vi "Vertical Profile.vi"(5 "Vert.Z-Locations":dbl[](array[numeric])=[12.7, 19.05, 25.4], 6 "Averaging time (min)":dbl, 7 "Starting Coords":T1={"X"=-100.0, "Y"=-150.0, "Z0"=45.0, "Name"="Anemo1"}, 10 "Tunnel Speed":dbl, 11 "Input Task Array":T4(array[cluster])) -> (3 "Output Task Array":T4(array[cluster]))   [LabVIEW 2015]
uses:
  Anemometry Sub Vis/Gen Trav/Spacing.ctl
  Anemometry Sub Vis/Controls/Multi_run_mode.ctl
  MRCMDFBGlobal.vi
  Set ADAM Ch.vi
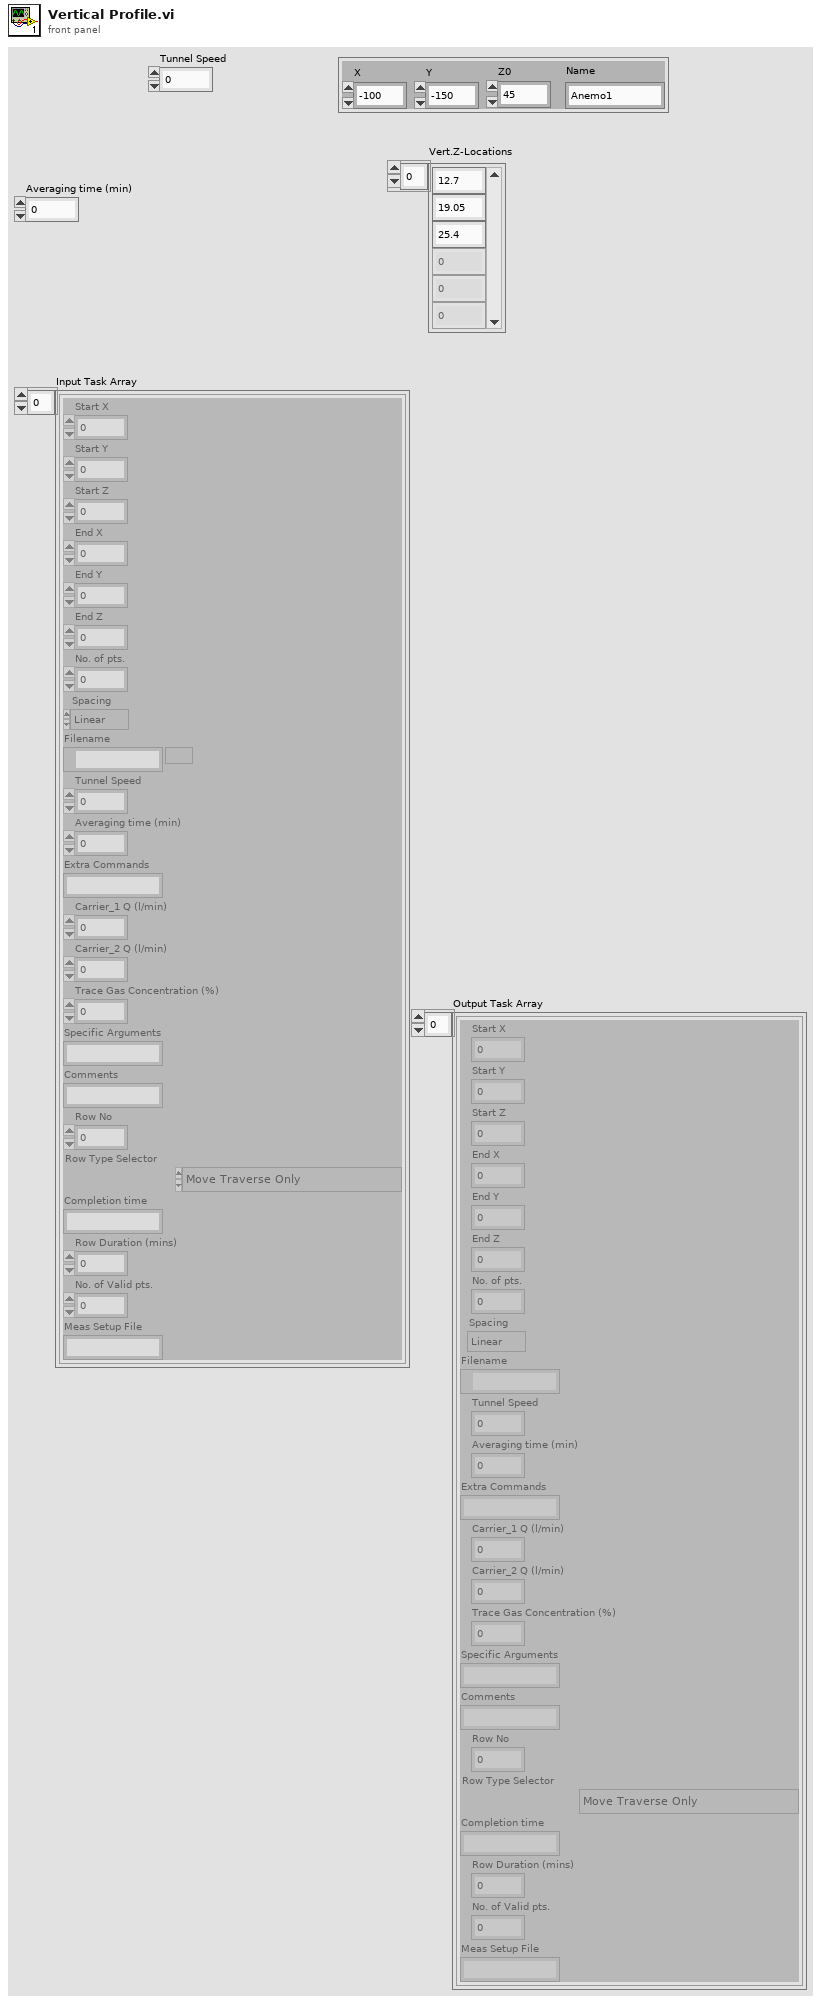
[diagram p1: front panel]
types:
  T1 = cluster{"X":dbl, "Y":dbl, "Z0":dbl, "Name":string}
  T2 = typedef "Spacing.ctl" = enum16{"Linear", "Log", "Gauss", "Specified", "N/A"}
  T3 = typedef "Multi_run_mode.ctl" = enum16{"Move Traverse Only", "Set Tunnel Speed Only", "Set Source Only", "Set Measurement Conditions", "Single Measurement", "Vertical Profile", "Lateral Profile", "Longitudinal Profile", "Explore Volume", "Multi-Axis Profile", "Auto Calibrate", "Meas Fast FID Bkgnd", "Check Beam Power", "Scanning Valve Measurement", "Run VI Named:", "Set ADAM Ch", "Wait (minutes)", "Send Message", "Synchronize With:", "Fall Back to this Row", "Turn Off Row Repeating", "Blank Row", "Traverse 3D Volume"}
  T4 = cluster{"Start X":sgl, "Start Y":sgl, "Start Z":sgl, "End X":sgl, "End Y":sgl, "End Z":sgl, "No. of pts.":i32, "Spacing":T2, "Filename":path, "Tunnel Speed":dbl, "Averaging time (min)":dbl, "Extra Commands":string, "Carrier_1 Q (l/min)":dbl, "Carrier_2 Q (l/min)":dbl, "Trace Gas Concentration (%)":dbl, "Specific Arguments":string, "Comments":string, "Row No":i32, "Row Type Selector":T3, "Completion time":string, "Row Duration (mins)":dbl, "No. of Valid pts.":i32, "Meas Setup File":string}[]
  T5 = cluster{"Start X":sgl, "Start Y":sgl, "Start Z":sgl, "End X":sgl, "End Y":sgl, "End Z":sgl, "No. of pts.":i32, "Spacing":T2, "Filename":path, "Tunnel Speed":dbl, "Averaging time (min)":dbl, "Extra Commands":string, "Carrier_1 Q (l/min)":dbl, "Carrier_2 Q (l/min)":dbl, "Trace Gas Concentration (%)":dbl, "Specific Arguments":string, "Comments":string, "Row No":i32, "Row Type Selector":T3, "Completion time":string, "Row Duration (mins)":dbl, "No. of Valid pts.":i32, "Meas Setup File":string}
  T6 = cluster{"Azimuth Array Index":u32, "Vert Prof Array Index":u32, "Lat Prof Array Index":u32, "Long Prof Array Index":u32}
  T7 = cluster{"TT.Azimuths":dbl[], "Z.HeightCorrs":dbl[][], "Use Height Corrections":bool, "Height Survey Filepaths":path[], "Corrections from File":bool}
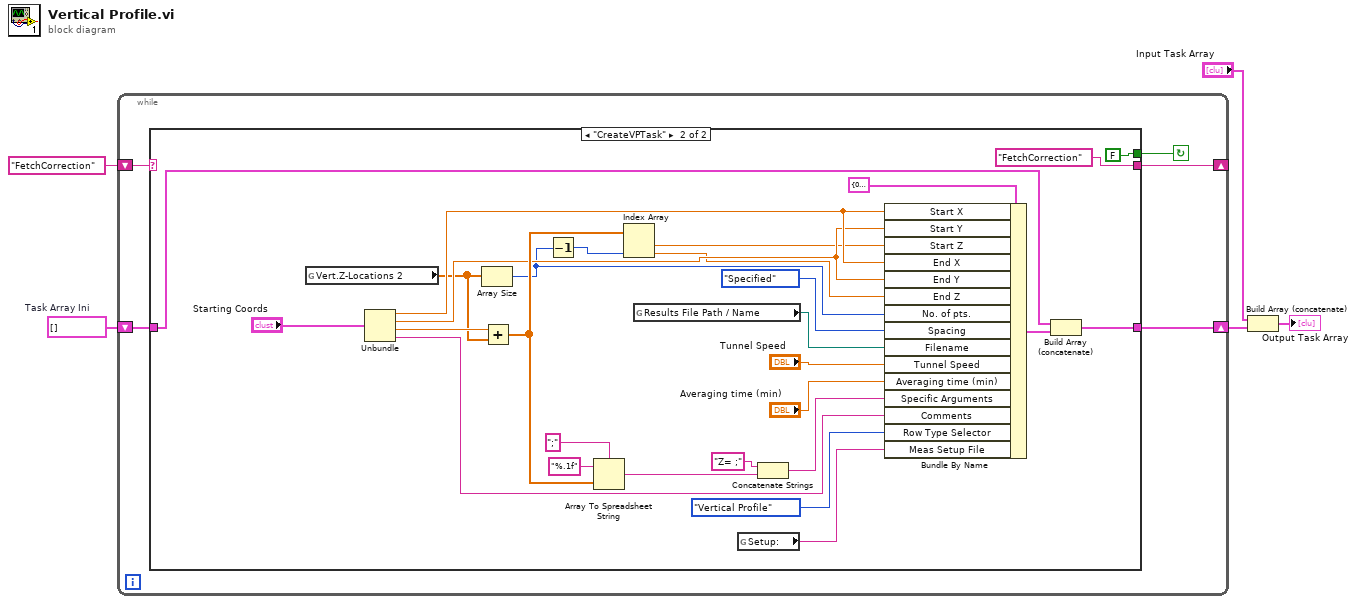
[diagram p0: block diagram]
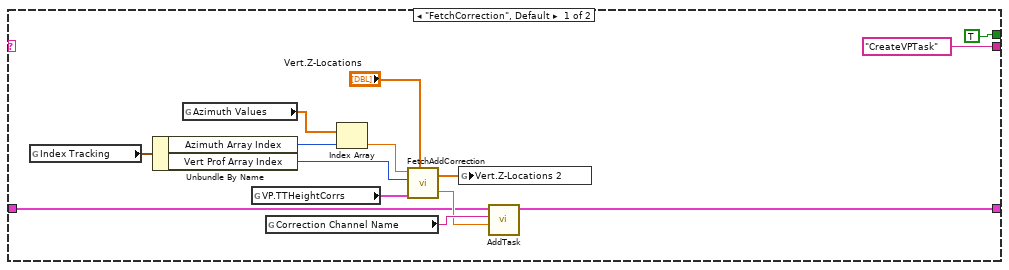
[diagram p2: hidden frame]
diagram:
  w1 = T4 []  # Task Array Ini
  n1 = while {
    shift-right: [w6] -> _
    shift-left: "FetchCorrection" -> [w9]
    shift-right: [w10] -> w3
    shift-left: w1 -> [w8]
    stop <- w7 continue-if-true
    n2 = case shown="\"CreateVPTask\"" w9 {
      tunnel: [w16 w28] -> w10
      tunnel: ["CreateVPTask" "FetchCorrection"] -> w6
      tunnel: w8 -> [w17 w27]
      tunnel: [TRUE FALSE] -> w7
      frame "FetchCorrection", Default {
        n3 = global read "MRCMDFBGlobal.vi" "Index Tracking"() -> (w22:T6)
        n4 = Unbundle By Name(w22) -> ("Azimuth Array Index"=w12:u32, "Vert Prof Array Index"=w21:u32)
        n5 = global read "MRCMDFBGlobal.vi" "Azimuth Values"() -> (w13:dbl[])
        n6 = global read "MRCMDFBGlobal.vi" "VP.TTHeightCorrs"() -> (w23:T7)
        n7 = global read "MRCMDFBGlobal.vi" "Correction Channel Name"() -> (w19:string)
        n8 = Index Array(array=w13, index=w12) -> (element=w11:dbl)
        n9 = call "FetchAddCorrection.vi"("Azimuth Value"=w11, "Vert Prof Array Index"=w21, "VP.TTHeightCorrs"=w23, "Vert.Z-Locations"="Vert.Z-Locations") -> ("Vert.Z-Locations 2"=w20:dbl[], "dz"=w18:dbl)  [unwired: 1 in]
        n10 = global write "MRCMDFBGlobal.vi" "Vert.Z-Locations 2"(w20) -> ()
        n11 = call-poly "AddTask.vi"("Value"=w18, "ADAM:Channel:Name"=w19, "Input Task Array"=w17) -> ("Output Task Array"=w16:T4)  [unwired: 8 in]
      }
      frame "CreateVPTask" {
        n12 = global read "MRCMDFBGlobal.vi" "Vert.Z-Locations 2"() -> (w25:dbl[])
        n13 = Unbundle("Starting Coords") -> ("X"=w38:dbl, "Y"=w37:dbl, "Z0"=w31:dbl, "Name"=w32:string)
        n14 = Array Size(array=w25) -> (size(s)=w35:i32)
        n15 = Add(x=w31, y=w25) -> (x+y=w45:dbl[])
        n16 = Decrement(x=w35) -> (x-1=w42:i32)
        n17 = Array To Spreadsheet String(delimiter (Tab)=";", array=w45, 3:"%.1f" ("format string")) -> (spreadsheet string=w43:string)
        n18 = Index Array(array=w45, index #2=w42) -> (element #1=w34:dbl, element #2=w33:dbl)  [unwired: 1 in]
        n19 = global read "MRCMDFBGlobal.vi" "Results File Path / Name"() -> (w46:path)
        n20 = global read "MRCMDFBGlobal.vi" "Setup:"() -> (w47:string)
        n21 = Concatenate Strings("Z= ;", w43) -> (w36:string)
        n22 = Bundle By Name(cluster=T5 {"Start X"=0.0, "Start Y"=0.0, "Start Z"=0.0, "End X"=0.0, "End Y"=0.0, "End Z"=0.0, "No. of pts."=0, "Spacing"=enum."Linear", "Filename"=path "", "Tunnel Speed"=0.0, "Averaging time (min)"=0.0, "Extra Commands"="", "Carrier_1 Q (l/min)"=0.0, "Carrier_2 Q (l/min)"=0.0, "Trace Gas Concentration (%)"=0.0, "Specific Arguments"="", "Comments"="", "Row No"=0, "Row Type Selector"=enum."Move Traverse Only", "Completion time"="", "Row Duration (mins)"=0.0, "No. of Valid pts."=0, "Meas Setup File"=""} ("RowTemplateConst"), "Start X"=w38, "Start Y"=w37, "Start Z"=w34, "End X"=w38, "End Y"=w37, "End Z"=w33, "No. of pts."=w35, "Spacing"=Spacing."Specified", "Filename"=w46, "Tunnel Speed"="Tunnel Speed", "Averaging time (min)"="Averaging time (min)", "Specific Arguments"=w36, "Comments"=w32, "Row Type Selector"=Multi_run_mode."Vertical Profile", "Meas Setup File"=w47) -> (w29:T5)
        n23 = Build Array (concatenate)(w27, w29) -> (w28:T4)
      }
    }
  }
  n24 = Build Array (concatenate)("Input Task Array", w3) -> (→"Output Task Array":T4)
